vi "Login.vi"(6 "passWord":string, 7 "remote port (21)":u16=21, 8 "error in (no error)":errorcluster, 9 "userName":string, 10 "address":string, 11 "FTP in":refnum<class "FTP.lvclass">) -> (0 "error out":errorcluster, 3 "FTP out":refnum<class "FTP.lvclass">)   [LabVIEW 2020, in "FTP.lvlib" / "FTP.lvclass"]
doc: "This vi will login to an ftp server using the Address, User Name, and Password. If no password is provided, then the vi will assume that one is not necessary to login."
uses:
  FTP.lvclass
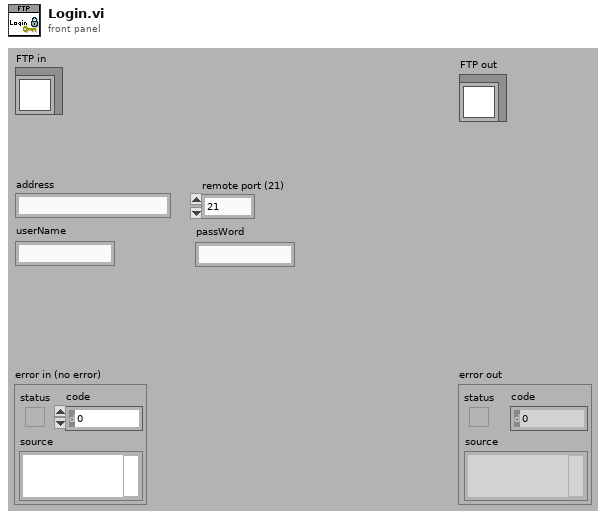
[diagram p1: front panel]
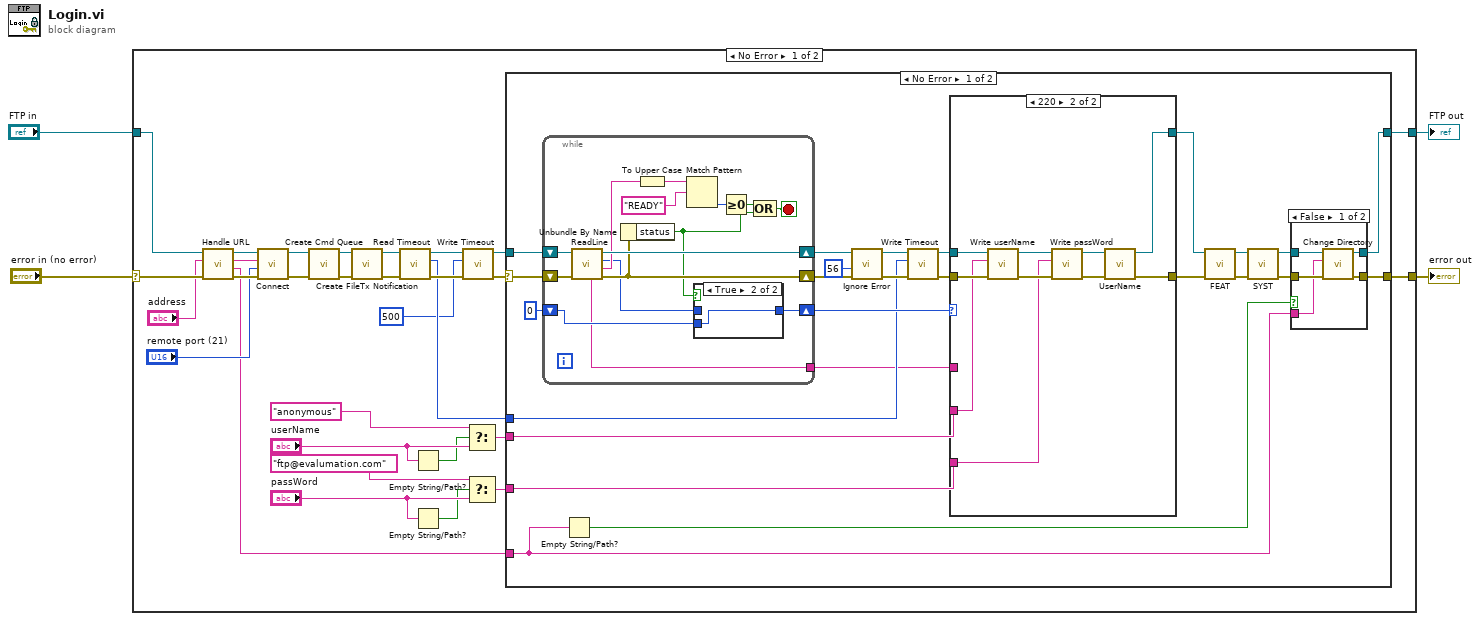
[diagram p0: block diagram]
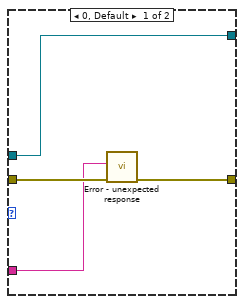
[diagram p4: hidden frame]
diagram:
  n1 = case shown="No Error" "error in (no error)" {
    selector: "error in (no error)" -> [w13 w100]
    tunnel: [w16 w100] -> w3
    tunnel: [w15 w99] -> w1
    tunnel: "FTP in" -> [w10 w99]
    frame No Error {
      n2 = call "Handle URL.vi"("error in (no error)"=w13, "URL"="address", "FTP in"=w10) -> ("error out"=w12:errorcluster, "directory"=w5:string, "address"=w8:string, "FTP out"=w11:refnum<class "FTP.lvclass">)  [unwired: 5 in]
      n3 = call "Connect.vi"("error in (no error)"=w12, "remote port (21)"="remote port (21)", "address"=w8, "FTP in"=w11) -> ("error out"=w33:errorcluster, "FTP out"=w34:refnum<class "FTP.lvclass">)  [unwired: 6 in]
      n4 = call "Create Cmd Queue.vi"("error in (no error)"=w33, "FTP in"=w34) -> ("error out"=w32:errorcluster, "FTP out"=w31:refnum<class "FTP.lvclass">)  [unwired: 8 in]
      n5 = call "Create FileTx Notification.vi"("error in (no error)"=w32, "FTP in"=w31) -> ("error out"=w22:errorcluster, "FTP out"=w23:refnum<class "FTP.lvclass">)  [unwired: 8 in]
      n6 = call "Read Timeout.vi"("error in (no error)"=w22, "FTP in"=w23) -> ("error out"=w20:errorcluster, "Timeout"=w18:i32, "FTP out"=w21:refnum<class "FTP.lvclass">)  [unwired: 7 in]
      n7 = Empty String/Path?(string/path="userName") -> (empty?=w29:bool)
      n8 = Empty String/Path?(string/path="passWord") -> (empty?=w24:bool)
      n9 = call "Write Timeout.vi"("error in (no error)"=w20, "Timeout"=500, "FTP in"=w21) -> ("error out"=w14:errorcluster, "FTP out"=w19:refnum<class "FTP.lvclass">)  [unwired: 7 in]
      n10 = Select(t="anonymous", s=w29, f="userName") -> (s? t:f=w28:string)
      n11 = Select(t="ftp@evalumation.com", s=w24, f="passWord") -> (s? t:f=w26:string)
      n12 = case shown="No Error" w14 {
        selector: w14 -> [w42 w97]
        tunnel: w28 -> [w55 _]
        tunnel: w26 -> [w54 _]
        tunnel: w19 -> [w50 w98]
        tunnel: w18 -> [w45 _]
        tunnel: [w39 w97] -> w16
        tunnel: [w37 w98] -> w15
        tunnel: w5 -> [w35 _]
        frame No Error {
          n13 = while {
            shift-right: [w80] -> w46
            shift-left: w50 -> [w79]
            shift-right: [w73] -> w53
            shift-left: w42 -> [w78]
            shift-right: [w69] -> w58
            shift-left: 0 ("code") -> [w67]
            tunnel: [w66] -> w41
            stop <- w71 stop-if-true
            n14 = call "ReadLine.vi"("error in (no error)"=w78, "FTP in"=w79) -> ("error out"=w73:errorcluster, "Line"=w74:string, "code"=w70:i32, "FTP out"=w80:refnum<class "FTP.lvclass">, "Full Line"=w66:string)  [unwired: 5 in]
            n15 = Unbundle By Name(w73) -> ("status"=w68:bool)
            n16 = To Upper Case(1:w74) -> (0:w76:string)
            n17 = Match Pattern(string=w76, regular expression="READY") -> (offset past match=w75:i32)  [unwired: 1 in, 3 out]
            n18 = case shown="True" w68 {
              tunnel: w70 -> [w81 _]
              tunnel: [w81 w82] -> w69
              tunnel: w67 -> [_ w82]
              frame False {
              }
              frame True {
              }
            }
            n19 = Greater Or Equal To 0?(x=w75) -> (x >= 0?=w72:bool)
            n20 = Compound Arithmetic op=OR(w72, w68) -> (w71:bool)
          }
          n21 = Empty String/Path?(string/path=w35) -> (empty?=w36:bool)
          n22 = call "Ignore Error.vi"("error in"=w53, "code"=56) -> ("error out"=w49:errorcluster)  [unwired: 9 in]
          n23 = call "Write Timeout.vi"("error in (no error)"=w49, "Timeout"=w45, "FTP in"=w46) -> ("error out"=w48:errorcluster, "FTP out"=w47:refnum<class "FTP.lvclass">)  [unwired: 7 in]
          n24 = case shown="220" w58 {
            tunnel: w48 -> [w85 w96]
            tunnel: w47 -> [w86 w91]
            tunnel: w55 -> [_ w90]
            tunnel: w54 -> [_ w89]
            tunnel: [w86 w88] -> w56
            tunnel: [w84 w87] -> w57
            tunnel: w41 -> [w83 _]
            frame 0, Default {
              n25 = call "Error - unexpected response.vi"("error in (no error)"=w85, "Full Response"=w83) -> ("error out"=w84:errorcluster)  [unwired: 9 in]
            }
            frame 220 {
              n26 = call "Write userName.vi"("error in (no error)"=w96, "userName"=w90, "FTP in"=w91) -> ("error out"=w95:errorcluster, "FTP out"=w92:refnum<class "FTP.lvclass">)  [unwired: 7 in]
              n27 = call "Write passWord.vi"("error in (no error)"=w95, "passWord"=w89, "FTP in"=w92) -> ("error out"=w94:errorcluster, "FTP out"=w93:refnum<class "FTP.lvclass">)  [unwired: 7 in]
              n28 = call "UserName.vi"("error in (no error)"=w94, "FTP in"=w93) -> ("error out"=w87:errorcluster, "FTP out"=w88:refnum<class "FTP.lvclass">)  [unwired: 8 in]
            }
          }
          n29 = call "FEAT.vi"("error in (no error)"=w57, "FTP in"=w56) -> ("error out"=w44:errorcluster, "FTP out"=w43:refnum<class "FTP.lvclass">)  [unwired: 8 in]
          n30 = call "SYST.vi"("error in (no error)"=w44, "FTP in"=w43) -> ("error out"=w40:errorcluster, "FTP out"=w38:refnum<class "FTP.lvclass">)  [unwired: 8 in]
          n31 = case shown="False" w36 {
            tunnel: w40 -> [w63 w64]
            tunnel: [w62 w64] -> w39
            tunnel: w38 -> [w61 w65]
            tunnel: [w60 w65] -> w37
            tunnel: w35 -> [w59 _]
            frame False {
              n32 = call "Change Directory.vi"("error in (no error)"=w63, "RemoteDirectory"=w59, "FTP in"=w61) -> ("error out"=w62:errorcluster, "FTP out"=w60:refnum<class "FTP.lvclass">)  [unwired: 7 in]
            }
            frame True {
            }
          }
        }
        frame Error {
        }
      }
    }
    frame Error {
    }
  }
  "error out" <- w3
  "FTP out" <- w1
